vi "integer_part_remover.vi"(0 "precision(2)":u8=2, 2 "numeric":dbl format="%#.13f") -> (6 "numeric string":string)   [LabVIEW 2025]
doc: "<b>numeric</b> is a floating point number: X.nnn...nnn, where X is any integer.\n<b>numeric string</b> will return an integer: nnn...nnn, where the number of decimal places is determined by <b>precision</b>."
panel:
  # "numeric is a floating point number: X.nnn...nnn, \nwhere X is any integer.\nnumeric string will return an integer: nnn...nnn, \nwhere the number of decimal places is determined \nby precision."
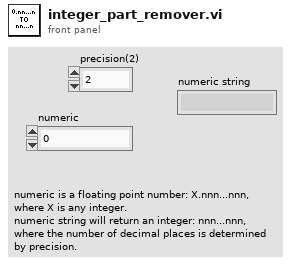
[diagram p1: front panel]
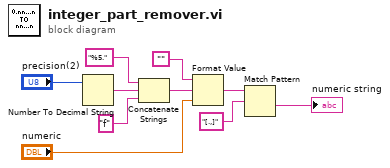
[diagram p0: block diagram]
diagram:
  n1 = Number To Decimal String(number="precision(2)") -> (decimal integer string=w1:string)  [unwired: 1 in]
  n2 = Concatenate Strings("%5." ("string"), w1, "f") -> (w3:string)
  n3 = Format Value(string ("")="", format string=w3, value (0)="numeric") -> (output string=w9:string)
  n4 = Match Pattern(string=w9, regular expression="[.,]") -> (after substring=→"numeric string":string)  [unwired: 1 in, 3 out]
